vi "Read Limit Volt.vi"(8 "error in":errorcluster, 11 "SimulatedPS in":refnum<class "SimulatedPS.lvclass">) -> (0 "error out":errorcluster, 2 "OverVolt_Protect":dbl, 3 "SimulatedPS out":refnum<class "SimulatedPS.lvclass">)   [LabVIEW 2019, in "SimulatedPS.lvlib" / "SimulatedPS.lvclass"]
uses:
  Library/SimulatedPS.lvclass
  builds/Instruments/PowerSupply.lvlibp/Library/PowerSupply.lvclass
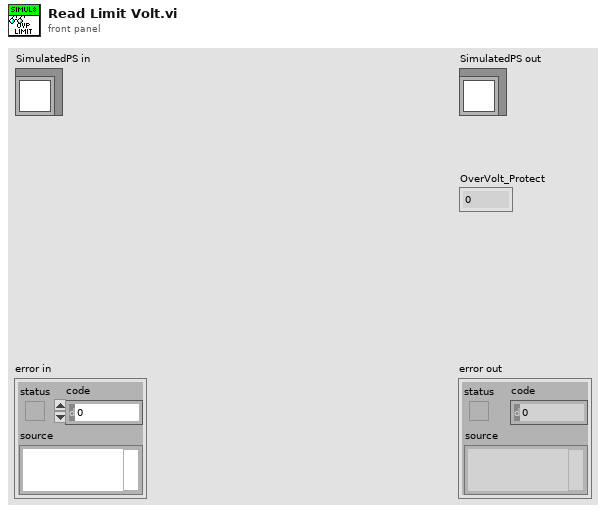
[diagram p1: front panel]
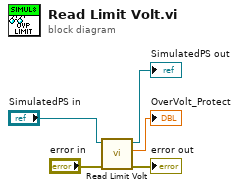
[diagram p0: block diagram]
diagram:
  n1 = call-parent "Read Limit Volt.vi"("error in"="error in", "PowerSupply in"="SimulatedPS in") -> ("error out"=→"error out":errorcluster, "OverVolt_Protect"=→"OverVolt_Protect":dbl, "PowerSupply out"=→"SimulatedPS out":refnum<class "SimulatedPS.lvclass">)  [unwired: 7 in]
